vi "标样核查.vi"() -> ()   [LabVIEW 2016, in "斯坦道多参数.lvlib"]
panel:
  out "运行状态":u16(ring) items=["空闲", "水样测试", "标样核查"]
  out "seconds since 1Jan1904":timestamp
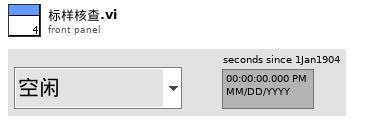
[diagram p1: front panel]
types:
  T1 = cluster{"ph":bool, "DO":bool, "Cond":bool, "Turb":bool, "叶绿素a":bool, "藻密度":bool, "ORP":bool, "cod":bool, "DO2":bool, "氯化物":bool, "氨氮":bool, "水中油":bool}
  T2 = cluster{"运行模式":enum16{"维护模式", "常规模式", "应急模式", "质控模式"}, "24H周期设置":bool[]}
  T3 = typedef "集成多参数单参数字段定义.ctl" = cluster{"时间":timestamp, "测量模式":string, "数据类型":string, "检测值":sgl, "单位":string, "数据标识":string, "标样参考值":sgl, "因子编码":string, "LastTime":timestamp}
  T4 = cluster{"数据保存间隔":dbl, "保存组数":dbl, "水温标样值":dbl, "pH标样值":dbl, "溶解氧标样值":dbl, "电导率标样值":dbl, "浊度标样值":dbl, "叶绿素a标样值":dbl, "藻密度标样值":dbl, "ORP标样值":dbl, "氯化物标样值":dbl, "COD标样值":dbl, "氨氮标样值":dbl, "水中油标样值":dbl, "pH启用":bool, "溶解氧启用":bool, "电导率启用":bool, "浊度启用":bool, "叶绿素a启用":bool, "藻密度启用":bool, "ORP启用":bool, "氯化物启用":bool, "COD启用":bool, "氨氮启用":bool, "水中油启用":bool}
  T5 = typedef "LVDateTimeRec.ctl" = cluster{"秒数的小数部分":dbl, "秒":i32, "分":i32, "时":i32, "日":i32, "月":i32, "年":i32, "天数（周）":i32, "天数（年）":i32, "DST":i32}
  T6 = cluster{"温度测量值":sgl, "测量值":sgl, "温度偏移修正值":sgl, "信号值":sgl, "数据标识":string}
  T7 = cluster{"温度测量值":sgl, "DO%":sgl, "DOmg/L":sgl, "温度偏移修正值":sgl, "数据标识mg/L":string, "数据标识%":string}
  T8 = cluster{"CH":u16, "监测值":dbl, "信号值":sgl, "数据标识":string}
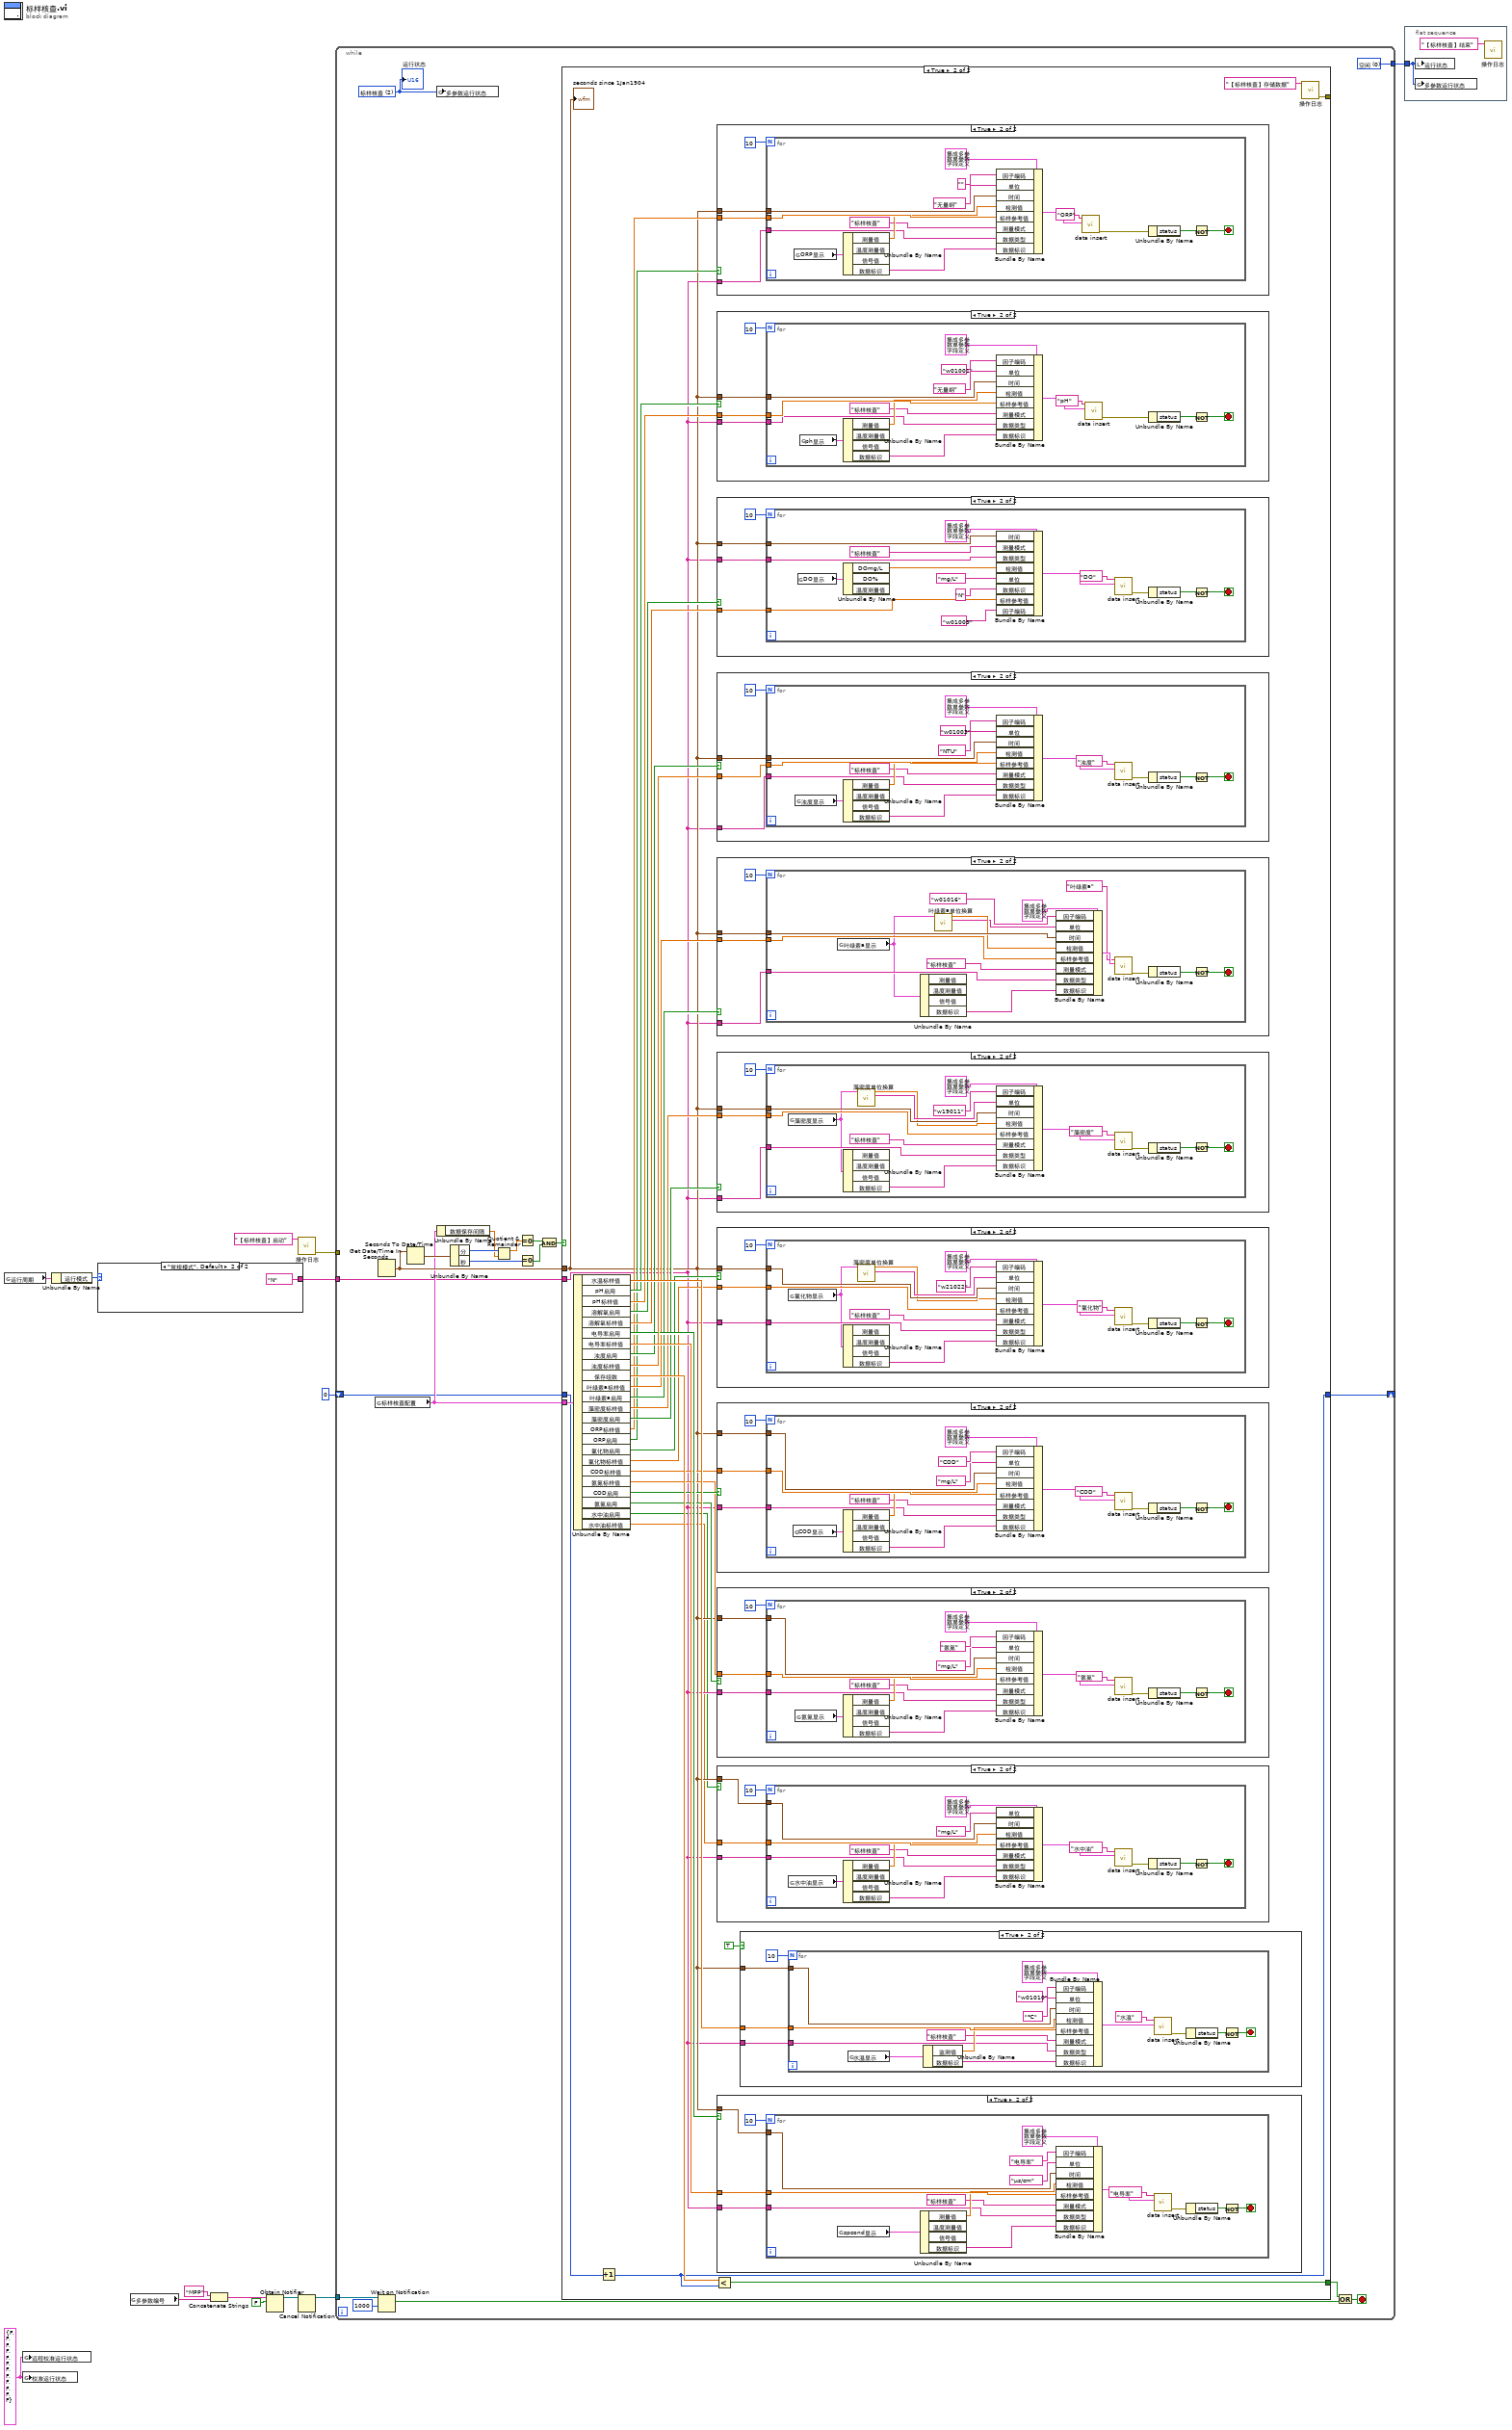
[diagram p0: block diagram]
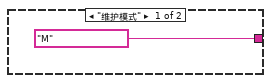
[diagram p2: hidden frame]
diagram:
  w1 = T1 {"ph"=FALSE, "DO"=FALSE, "Cond"=FALSE, "Turb"=FALSE, "叶绿素a"=FALSE, "藻密度"=FALSE, "ORP"=FALSE, "cod"=FALSE, "DO2"=FALSE, "氯化物"=FALSE, "氨氮"=FALSE, "水中油"=FALSE} ("远程校准运行状态")
  n1 = global read "断电保存变量.vi" "运行周期"() -> (w3:T2)
  n2 = global write "多参数全局变量.vi" "远程校准运行状态"(w1) -> ()
  n3 = global write "多参数全局变量.vi" "校准运行状态"(w1) -> ()
  n4 = Unbundle By Name(w3) -> ("运行模式"=w2:enum16{"维护模式", "常规模式", "应急模式", "质控模式"})
  n5 = case shown="\"常规模式\", Default" w2 {
    tunnel: ["M" ("数据标记表") "N" ("数据标记表")] -> w4
    frame "维护模式" {
    }
    frame "常规模式", Default {
    }
  }
  n6 = global read "多参数全局变量.vi" "多参数编号"() -> (w8:string)
  n7 = Concatenate Strings("MPP" ("名称（未命名）"), w8) -> (w9:string)
  n8 = Obtain Notifier(name (unnamed)=w9, notification data type=FALSE) -> (notifier out=w12:refnum<notifier>)  [unwired: 2 in, 2 out]
  n9 = call "操作日志.vi"("日志信息"="【标样核查】启动") -> ("error out"=w6:errorcluster)  [unwired: 10 in]
  n10 = Cancel Notification(0:w12) -> (8:w11:refnum<notifier>)  [unwired: 1 in, 2 out]
  n11 = while {
    tunnel: [w27] -> w10
    tunnel: w11 -> [w26]
    tunnel: w6 -> [_]
    shift-right: [w20] -> _
    shift-left: 0 -> [w21]
    tunnel: w4 -> [w17]
    stop <- w19 stop-if-true
    w27 = u16 0 items=["空闲", "水样测试", "标样核查"] ("多参数运行状态")
    w23 = u16 2 items=["空闲", "水样测试", "标样核查"] ("多参数运行状态")
    n12 = global read "断电保存变量.vi" "标样核查配置"() -> (w22:T4)
    n13 = Get Date/Time In Seconds() -> (seconds since 1Jan1904=w28:timestamp)
    n14 = Wait on Notification(notifier=w26, timeout in ms (-1)=1000 ("超时毫秒(-1)")) -> (notification=w24:bool)  [unwired: 2 in, 3 out]
    n15 = Seconds To Date/Time(time stamp (now)=w28) -> (date time rec=w36:T5)  [unwired: 1 in]
    n16 = global write "多参数全局变量.vi" "多参数运行状态"(w23) -> ()
    n17 = Unbundle By Name(w22) -> ("数据保存间隔"=w31:dbl)
    n18 = Unbundle By Name(w36) -> ("分"=w32:i32, "秒"=w35:i32)
    n19 = Quotient & Remainder(x=w32, y=w31) -> (x-y*floor(x/y)=w30:dbl)  [unwired: 1 out]
    n20 = Equal To 0?(x=w30) -> (x = 0?=w29:bool)
    n21 = Equal To 0?(x=w35) -> (x = 0?=w34:bool)
    n22 = And(x=w29, y=w34) -> (x .and. y?=w33:bool)
    n23 = case shown="True" w33 {
      tunnel: w22 -> [_ w70]
      tunnel: w28 -> [_ w41]
      tunnel: [_ w63] -> _
      tunnel: w21 -> [w37 w57]
      tunnel: [w37 w55] -> w20
      tunnel: [_ w54] -> w18
      tunnel: w17 -> [_ w40]
      frame False {
      }
      frame True {
        n24 = Unbundle By Name(w70) -> ("水温标样值"=w69:dbl, "pH启用"=w62:bool, "pH标样值"=w68:dbl, "溶解氧启用"=w60:bool, "溶解氧标样值"=w67:dbl, "电导率启用"=w59:bool, "电导率标样值"=w66:dbl, "浊度启用"=w58:bool, "浊度标样值"=w65:dbl, "保存组数"=w56:dbl, "叶绿素a标样值"=w53:dbl, "叶绿素a启用"=w50:bool, "藻密度标样值"=w52:dbl, "藻密度启用"=w51:bool, "ORP标样值"=w49:dbl, "ORP启用"=w48:bool, "氯化物启用"=w47:bool, "氯化物标样值"=w46:dbl, "COD标样值"=w44:dbl, "氨氮标样值"=w42:dbl, "COD启用"=w45:bool, "氨氮启用"=w43:bool, "水中油启用"=w38:bool, "水中油标样值"=w39:dbl)
        n25 = Increment(x=w57) -> (x+1=w55:i32)
        n26 = Less?(x=w56, y=w55) -> (x < y?=w54:bool)
        n27 = case shown="True" w48 {
          tunnel: w49 -> [_ w149]
          tunnel: w41 -> [_ w147]
          tunnel: w40 -> [_ w146]
          frame False {
          }
          frame True {
            n28 = for {
              N: 10 -> [_]
              tunnel: w149 -> [w163]
              tunnel: w147 -> [w157]
              tunnel: w146 -> [w153]
              stop <- w158 stop-if-true
              n29 = global read "多参数全局变量.vi" "ORP显示"() -> (w162:T6)
              n30 = Unbundle By Name(w162) -> ("测量值"=w161:sgl, "数据标识"=w154:string)  [unwired: 2 out]
              n31 = Bundle By Name(cluster=T3 {"时间"=timestamp(0 s since 1904-01-01), "测量模式"="水样测试", "数据类型"="N", "检测值"=0.0, "单位"="mg/L", "数据标识"="N", "标样参考值"=0.0, "因子编码"="", "LastTime"=timestamp(0 s since 1904-01-01)} ("data"), "因子编码"="", "单位"="无量纲", "时间"=w157, "检测值"=w161, "标样参考值"=w163, "测量模式"="标样核查", "数据类型"=w153, "数据标识"=w154) -> (w156:T3)
              n32 = call "data insert.vi"("data"=w156, "table in"="ORP") -> ("error out"=w160:errorcluster)  [unwired: 9 in]
              n33 = Unbundle By Name(w160) -> ("status"=w159:bool)
              n34 = Not(x=w159) -> (.not. x?=w158:bool)
            }
          }
        }
        n35 = case shown="True" w62 {
          tunnel: w68 -> [_ w263]
          tunnel: w41 -> [_ w261]
          tunnel: w40 -> [_ w260]
          frame False {
          }
          frame True {
            n36 = for {
              N: 10 -> [_]
              tunnel: w263 -> [w275]
              tunnel: w261 -> [w269]
              tunnel: w260 -> [w265]
              stop <- w270 stop-if-true
              n37 = global read "多参数全局变量.vi" "ph显示"() -> (w274:T6)
              n38 = Unbundle By Name(w274) -> ("测量值"=w273:sgl, "数据标识"=w266:string)  [unwired: 2 out]
              n39 = Bundle By Name(cluster=T3 {"时间"=timestamp(0 s since 1904-01-01), "测量模式"="水样测试", "数据类型"="N", "检测值"=0.0, "单位"="mg/L", "数据标识"="N", "标样参考值"=0.0, "因子编码"="", "LastTime"=timestamp(0 s since 1904-01-01)} ("data"), "因子编码"="w01001", "单位"="无量纲", "时间"=w269, "检测值"=w273, "标样参考值"=w275, "测量模式"="标样核查", "数据类型"=w265, "数据标识"=w266) -> (w268:T3)
              n40 = call "data insert.vi"("data"=w268, "table in"="pH" ("table输入")) -> ("error out"=w272:errorcluster)  [unwired: 9 in]
              n41 = Unbundle By Name(w272) -> ("status"=w271:bool)
              n42 = Not(x=w271) -> (.not. x?=w270:bool)
            }
          }
        }
        n43 = case shown="True" w60 {
          tunnel: w67 -> [_ w244]
          tunnel: w41 -> [_ w242]
          tunnel: w40 -> [_ w241]
          frame False {
          }
          frame True {
            n44 = for {
              N: 10 -> [_]
              tunnel: w244 -> [w249]
              tunnel: w242 -> [w254]
              tunnel: w241 -> [w246]
              stop <- w257 stop-if-true
              n45 = global read "多参数全局变量.vi" "DO显示"() -> (w259:T7)
              n46 = Unbundle By Name(w259) -> ("DOmg/L"=w252:sgl)  [unwired: 2 out]
              n47 = Bundle By Name(cluster=T3 {"时间"=timestamp(0 s since 1904-01-01), "测量模式"="水样测试", "数据类型"="N", "检测值"=0.0, "单位"="mg/L", "数据标识"="N", "标样参考值"=0.0, "因子编码"="", "LastTime"=timestamp(0 s since 1904-01-01)} ("data"), "时间"=w254, "测量模式"="标样核查", "数据类型"=w246, "检测值"=w252, "单位"="mg/L", "数据标识"="N" ("水样数据标识"), "标样参考值"=w249, "因子编码"="w01009") -> (w255:T3)
              n48 = call "data insert.vi"("data"=w255, "table in"="DO") -> ("error out"=w247:errorcluster)  [unwired: 9 in]
              n49 = Unbundle By Name(w247) -> ("status"=w258:bool)
              n50 = Not(x=w258) -> (.not. x?=w257:bool)
            }
          }
        }
        n51 = case shown="True" w58 {
          tunnel: w65 -> [_ w206]
          tunnel: w41 -> [_ w204]
          tunnel: w40 -> [_ w203]
          frame False {
          }
          frame True {
            n52 = for {
              N: 10 -> [_]
              tunnel: w206 -> [w217]
              tunnel: w204 -> [w211]
              tunnel: w203 -> [w208]
              stop <- w212 stop-if-true
              n53 = global read "多参数全局变量.vi" "浊度显示"() -> (w216:T6)
              n54 = Unbundle By Name(w216) -> ("测量值"=w215:sgl, "数据标识"=w209:string)  [unwired: 2 out]
              n55 = Bundle By Name(cluster=T3 {"时间"=timestamp(0 s since 1904-01-01), "测量模式"="水样测试", "数据类型"="N", "检测值"=0.0, "单位"="mg/L", "数据标识"="N", "标样参考值"=0.0, "因子编码"="", "LastTime"=timestamp(0 s since 1904-01-01)} ("data"), "因子编码"="w01003", "单位"="NTU", "时间"=w211, "检测值"=w215, "标样参考值"=w217, "测量模式"="标样核查", "数据类型"=w208, "数据标识"=w209) -> (w220:T3)
              n56 = call "data insert.vi"("data"=w220, "table in"="浊度" ("table输入")) -> ("error out"=w214:errorcluster)  [unwired: 9 in]
              n57 = Unbundle By Name(w214) -> ("status"=w213:bool)
              n58 = Not(x=w213) -> (.not. x?=w212:bool)
            }
          }
        }
        n59 = case shown="True" w50 {
          tunnel: w53 -> [_ w187]
          tunnel: w41 -> [_ w185]
          tunnel: w40 -> [_ w184]
          frame False {
          }
          frame True {
            n60 = for {
              N: 10 -> [_]
              tunnel: w187 -> [w199]
              tunnel: w185 -> [w195]
              tunnel: w184 -> [w192]
              stop <- w196 stop-if-true
              n61 = global read "多参数全局变量.vi" "叶绿素a显示"() -> (w190:T6)
              n62 = Unbundle By Name(w190) -> ("数据标识"=w193:string)  [unwired: 3 out]
              n63 = call "叶绿素a单位换算.vi"("叶绿素a显示"=w190) -> ("检测值1.单位"=w188:string, "测量值"=w189:sgl)  [unwired: 8 in, 1 out]
              n64 = Bundle By Name(cluster=T3 {"时间"=timestamp(0 s since 1904-01-01), "测量模式"="水样测试", "数据类型"="N", "检测值"=0.0, "单位"="mg/L", "数据标识"="N", "标样参考值"=0.0, "因子编码"="", "LastTime"=timestamp(0 s since 1904-01-01)} ("data"), "因子编码"="w01016", "单位"=w188, "时间"=w195, "检测值"=w189, "标样参考值"=w199, "测量模式"="标样核查", "数据类型"=w192, "数据标识"=w193) -> (w202:T3)
              n65 = call "data insert.vi"("data"=w202, "table in"="叶绿素a" ("table输入")) -> ("error out"=w198:errorcluster)  [unwired: 9 in]
              n66 = Unbundle By Name(w198) -> ("status"=w197:bool)
              n67 = Not(x=w197) -> (.not. x?=w196:bool)
            }
          }
        }
        n68 = case shown="True" w51 {
          tunnel: w52 -> [_ w168]
          tunnel: w41 -> [_ w166]
          tunnel: w40 -> [_ w165]
          frame False {
          }
          frame True {
            n69 = for {
              N: 10 -> [_]
              tunnel: w168 -> [w180]
              tunnel: w166 -> [w176]
              tunnel: w165 -> [w173]
              stop <- w177 stop-if-true
              n70 = global read "多参数全局变量.vi" "藻密度显示"() -> (w171:T6)
              n71 = Unbundle By Name(w171) -> ("数据标识"=w174:string)  [unwired: 3 out]
              n72 = call "藻密度单位换算.vi"("藻密度显示"=w171) -> ("检测值1.单位"=w170:string, "测量值"=w169:sgl)  [unwired: 8 in, 1 out]
              n73 = Bundle By Name(cluster=T3 {"时间"=timestamp(0 s since 1904-01-01), "测量模式"="水样测试", "数据类型"="N", "检测值"=0.0, "单位"="mg/L", "数据标识"="N", "标样参考值"=0.0, "因子编码"="", "LastTime"=timestamp(0 s since 1904-01-01)} ("data"), "因子编码"="w19011", "单位"=w170, "时间"=w176, "检测值"=w169, "标样参考值"=w180, "测量模式"="标样核查", "数据类型"=w173, "数据标识"=w174) -> (w183:T3)
              n74 = call "data insert.vi"("data"=w183, "table in"="藻密度" ("table输入")) -> ("error out"=w179:errorcluster)  [unwired: 9 in]
              n75 = Unbundle By Name(w179) -> ("status"=w178:bool)
              n76 = Not(x=w178) -> (.not. x?=w177:bool)
            }
          }
        }
        n77 = case shown="True" w47 {
          tunnel: w46 -> [_ w130]
          tunnel: w41 -> [_ w128]
          tunnel: w40 -> [_ w127]
          frame False {
          }
          frame True {
            n78 = for {
              N: 10 -> [_]
              tunnel: w130 -> [w144]
              tunnel: w128 -> [w140]
              tunnel: w127 -> [w137]
              stop <- w141 stop-if-true
              n79 = global read "多参数全局变量.vi" "氯化物显示"() -> (w135:T6)
              n80 = Unbundle By Name(w135) -> ("数据标识"=w138:string)  [unwired: 3 out]
              n81 = call "藻密度单位换算.vi"("藻密度显示"=w135) -> ("检测值1.单位"=w134:string, "测量值"=w133:sgl)  [unwired: 8 in, 1 out]
              n82 = Bundle By Name(cluster=T3 {"时间"=timestamp(0 s since 1904-01-01), "测量模式"="水样测试", "数据类型"="N", "检测值"=0.0, "单位"="mg/L", "数据标识"="N", "标样参考值"=0.0, "因子编码"="", "LastTime"=timestamp(0 s since 1904-01-01)} ("data"), "因子编码"="w21022", "单位"=w134, "时间"=w140, "检测值"=w133, "标样参考值"=w144, "测量模式"="标样核查", "数据类型"=w137, "数据标识"=w138) -> (w145:T3)
              n83 = call "data insert.vi"("data"=w145, "table in"="氯化物") -> ("error out"=w143:errorcluster)  [unwired: 9 in]
              n84 = Unbundle By Name(w143) -> ("status"=w142:bool)
              n85 = Not(x=w142) -> (.not. x?=w141:bool)
            }
          }
        }
        n86 = case shown="True" w45 {
          tunnel: w44 -> [_ w111]
          tunnel: w41 -> [_ w109]
          tunnel: w40 -> [_ w108]
          frame False {
          }
          frame True {
            n87 = for {
              N: 10 -> [_]
              tunnel: w111 -> [w123]
              tunnel: w109 -> [w117]
              tunnel: w108 -> [w113]
              stop <- w118 stop-if-true
              n88 = global read "多参数全局变量.vi" "COD显示"() -> (w122:T6)
              n89 = Unbundle By Name(w122) -> ("测量值"=w121:sgl, "数据标识"=w114:string)  [unwired: 2 out]
              n90 = Bundle By Name(cluster=T3 {"时间"=timestamp(0 s since 1904-01-01), "测量模式"="水样测试", "数据类型"="N", "检测值"=0.0, "单位"="mg/L", "数据标识"="N", "标样参考值"=0.0, "因子编码"="", "LastTime"=timestamp(0 s since 1904-01-01)} ("data"), "因子编码"="COD", "单位"="mg/L", "时间"=w117, "检测值"=w121, "标样参考值"=w123, "测量模式"="标样核查", "数据类型"=w113, "数据标识"=w114) -> (w126:T3)
              n91 = call "data insert.vi"("data"=w126, "table in"="COD" ("table输入")) -> ("error out"=w120:errorcluster)  [unwired: 9 in]
              n92 = Unbundle By Name(w120) -> ("status"=w119:bool)
              n93 = Not(x=w119) -> (.not. x?=w118:bool)
            }
          }
        }
        n94 = case shown="True" w43 {
          tunnel: w42 -> [_ w92]
          tunnel: w41 -> [_ w90]
          tunnel: w40 -> [_ w89]
          frame False {
          }
          frame True {
            n95 = for {
              N: 10 -> [_]
              tunnel: w92 -> [w104]
              tunnel: w90 -> [w98]
              tunnel: w89 -> [w94]
              stop <- w99 stop-if-true
              n96 = global read "多参数全局变量.vi" "氨氮显示"() -> (w103:T6)
              n97 = Unbundle By Name(w103) -> ("测量值"=w102:sgl, "数据标识"=w95:string)  [unwired: 2 out]
              n98 = Bundle By Name(cluster=T3 {"时间"=timestamp(0 s since 1904-01-01), "测量模式"="水样测试", "数据类型"="N", "检测值"=0.0, "单位"="mg/L", "数据标识"="N", "标样参考值"=0.0, "因子编码"="", "LastTime"=timestamp(0 s since 1904-01-01)} ("data"), "因子编码"="氨氮", "单位"="mg/L", "时间"=w98, "检测值"=w102, "标样参考值"=w104, "测量模式"="标样核查", "数据类型"=w94, "数据标识"=w95) -> (w107:T3)
              n99 = call "data insert.vi"("data"=w107, "table in"="氨氮" ("table输入")) -> ("error out"=w101:errorcluster)  [unwired: 9 in]
              n100 = Unbundle By Name(w101) -> ("status"=w100:bool)
              n101 = Not(x=w100) -> (.not. x?=w99:bool)
            }
          }
        }
        n102 = case shown="True" w38 {
          tunnel: w39 -> [_ w74]
          tunnel: w41 -> [_ w72]
          tunnel: w40 -> [_ w71]
          frame False {
          }
          frame True {
            n103 = for {
              N: 10 -> [_]
              tunnel: w74 -> [w86]
              tunnel: w72 -> [w80]
              tunnel: w71 -> [w76]
              stop <- w81 stop-if-true
              n104 = global read "多参数全局变量.vi" "水中油显示"() -> (w85:T6)
              n105 = Unbundle By Name(w85) -> ("测量值"=w84:sgl, "数据标识"=w77:string)  [unwired: 2 out]
              n106 = Bundle By Name(cluster=T3 {"时间"=timestamp(0 s since 1904-01-01), "测量模式"="水样测试", "数据类型"="N", "检测值"=0.0, "单位"="mg/L", "数据标识"="N", "标样参考值"=0.0, "因子编码"="", "LastTime"=timestamp(0 s since 1904-01-01)} ("data"), "单位"="mg/L", "时间"=w80, "检测值"=w84, "标样参考值"=w86, "测量模式"="标样核查", "数据类型"=w76, "数据标识"=w77) -> (w88:T3)
              n107 = call "data insert.vi"("data"=w88, "table in"="水中油" ("table输入")) -> ("error out"=w83:errorcluster)  [unwired: 9 in]
              n108 = Unbundle By Name(w83) -> ("status"=w82:bool)
              n109 = Not(x=w82) -> (.not. x?=w81:bool)
            }
          }
        }
        n110 = case shown="True" w59 {
          tunnel: w66 -> [_ w225]
          tunnel: w41 -> [_ w223]
          tunnel: w40 -> [_ w222]
          frame False {
          }
          frame True {
            n111 = for {
              N: 10 -> [_]
              tunnel: w225 -> [w237]
              tunnel: w223 -> [w231]
              tunnel: w222 -> [w227]
              stop <- w232 stop-if-true
              n112 = global read "多参数全局变量.vi" "spcond显示"() -> (w236:T6)
              n113 = Unbundle By Name(w236) -> ("测量值"=w235:sgl, "数据标识"=w228:string)  [unwired: 2 out]
              n114 = Bundle By Name(cluster=T3 {"时间"=timestamp(0 s since 1904-01-01), "测量模式"="水样测试", "数据类型"="N", "检测值"=0.0, "单位"="mg/L", "数据标识"="N", "标样参考值"=0.0, "因子编码"="", "LastTime"=timestamp(0 s since 1904-01-01)} ("data"), "因子编码"="电导率", "单位"="μs/cm", "时间"=w231, "检测值"=w235, "标样参考值"=w237, "测量模式"="标样核查", "数据类型"=w227, "数据标识"=w228) -> (w240:T3)
              n115 = call "data insert.vi"("data"=w240, "table in"="电导率" ("table输入")) -> ("error out"=w234:errorcluster)  [unwired: 9 in]
              n116 = Unbundle By Name(w234) -> ("status"=w233:bool)
              n117 = Not(x=w233) -> (.not. x?=w232:bool)
            }
          }
        }
        n118 = case shown="True" TRUE {
          tunnel: w69 -> [_ w282]
          tunnel: w41 -> [_ w281]
          tunnel: w40 -> [_ w279]
          frame False {
          }
          frame True {
            n119 = for {
              N: 10 -> [_]
              tunnel: w282 -> [w293]
              tunnel: w281 -> [w290]
              tunnel: w279 -> [w284]
              stop <- w287 stop-if-true
              n120 = global read "多参数全局变量.vi" "水温显示"() -> (w292:T8)
              n121 = Unbundle By Name(w292) -> ("监测值"=w291:dbl, "数据标识"=w285:string)
              n122 = Bundle By Name(cluster=T3 {"时间"=timestamp(0 s since 1904-01-01), "测量模式"="水样测试", "数据类型"="N", "检测值"=0.0, "单位"="mg/L", "数据标识"="N", "标样参考值"=0.0, "因子编码"="", "LastTime"=timestamp(0 s since 1904-01-01)} ("data"), "因子编码"="w01010", "单位"="℃", "时间"=w290, "检测值"=w291, "标样参考值"=w293, "测量模式"="标样核查", "数据类型"=w284, "数据标识"=w285) -> (w296:T3)
              n123 = call "data insert.vi"("data"=w296, "table in"="水温" ("table输入")) -> ("error out"=w289:errorcluster)  [unwired: 9 in]
              n124 = Unbundle By Name(w289) -> ("status"=w288:bool)
              n125 = Not(x=w288) -> (.not. x?=w287:bool)
            }
          }
        }
        n126 = call "操作日志.vi"("日志信息"="【标样核查】存储数据") -> ("error out"=w63:errorcluster)  [unwired: 10 in]
        "seconds since 1Jan1904" <- w41
      }
    }
    n127 = Or(x=w18, y=w24) -> (x .or. y?=w19:bool)
    "运行状态" <- w23
  }
  n128 = flat-sequence {
    tunnel: w10 -> [w299]
    frame #0 {
      n129 = local write "运行状态"(w299) -> ()
      n130 = global write "多参数全局变量.vi" "多参数运行状态"(w299) -> ()
      n131 = call "操作日志.vi"("日志信息"="【标样核查】结束") -> ()  [unwired: 10 in, 1 out]
    }
  }
